vi "Get Errors.vi"(8 "error in (no error)":errorcluster, 10 "Parse All":bool, 11 "Plugin Manager in":refnum<class "CIFPluginManager.lvclass">) -> (0 "error out":errorcluster, 2 "Errors":T1[](array[typedef]), 3 "Plugin Manager out":refnum<class "CIFPluginManager.lvclass">)   [LabVIEW 2021, in "CIFPluginManager.lvclass"]
uses:
  CIFPluginManager.lvclass
  <vilib>/CIF Foundation/CIF Core/CIFUtilities/CIFLogs/Typedef/Error Message.ctl
  CIFPluginManager.lvclass/CIFPluginManager.ctl
  <vilib>/CIF Foundation/CIF Core/CIFUtilities/CIFLogs/CIFLogs.lvlib
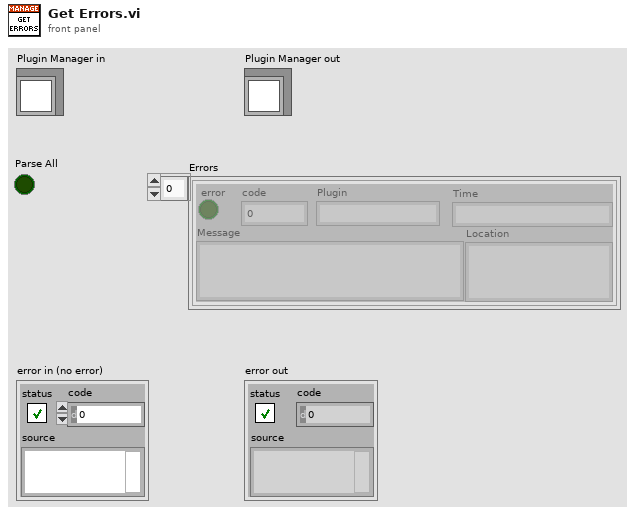
[diagram p1: front panel]
types:
  T1 = typedef "CIFLogs.lvlib/Error Message.ctl" = cluster{"error":bool, "code":i32, "Message":string, "Location":string, "Plugin":string, "Time":string}
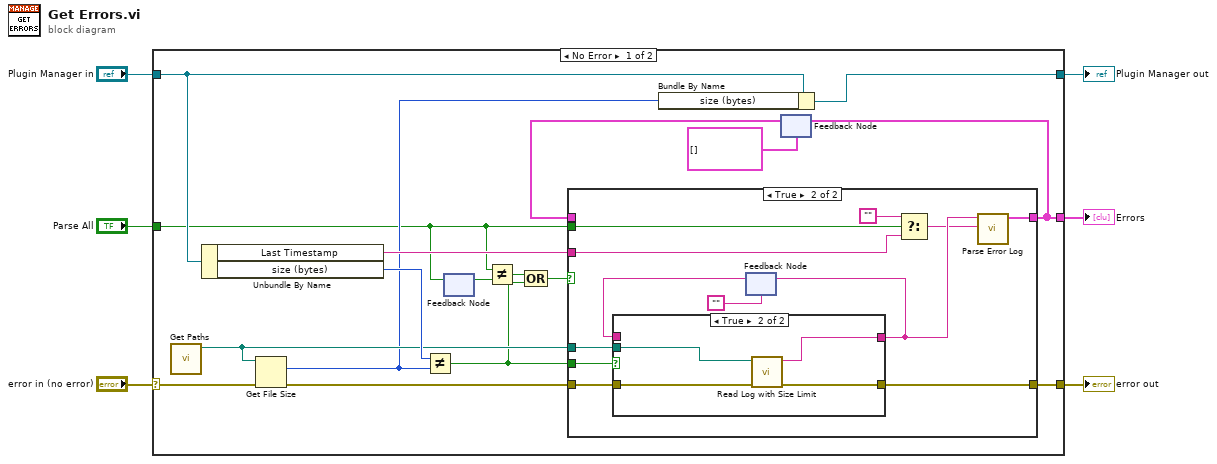
[diagram p0: block diagram]
diagram:
  n1 = case shown="No Error" "error in (no error)" {
    selector: "error in (no error)" -> [w18 w45]
    tunnel: [w23 w45] -> w1
    tunnel: [w19 w44] -> w3
    tunnel: "Plugin Manager in" -> [w20 w44]
    tunnel: [w9 _] -> w2
    tunnel: "Parse All" -> [w13 _]
    frame No Error {
      n2 = call <vilib>:"Get Paths.vi"() -> ("Error Log"=w17:path)  [unwired: 9 in, 2 out]
      n3 = Unbundle By Name(w20) -> ("Last Timestamp"=w21:string, "size (bytes)"=w22:i64)
      n4 = Get File Size(file=w17, error in=w18) -> (size (in bytes)=w15:i64, 0:w16:errorcluster)  [unwired: 1 out]
      n5 = Not Equal?(x=w22, y=w15) -> (x != y?=w11:bool)
      n6 = feedback-in #1(w13) -> ()
      n7 = feedback #1() -> (w14:bool)  [unwired: 1 in]
      n8 = Not Equal?(x=w13, y=w14) -> (x != y?=w12:bool)
      n9 = Compound Arithmetic op=OR(w12, w11) -> (w10:bool)
      n10 = Bundle By Name(cluster=w20, "size (bytes)"=w15) -> (w19:refnum<class "CIFPluginManager.lvclass">)
      n11 = feedback #2(T1[] [] ("Errors")) -> (w8:T1[])
      n12 = case shown="True" w10 {
        tunnel: [w24 w37] -> w23
        tunnel: [w25 w31] -> w9
        tunnel: w21 -> [_ w30]
        tunnel: w17 -> [_ w29]
        tunnel: w16 -> [w24 w28]
        tunnel: w13 -> [_ w27]
        tunnel: w11 -> [_ w26]
        tunnel: w8 -> [w25 _]
        frame False {
        }
        frame True {
          n13 = feedback #3("") -> (w34:string)
          n14 = case shown="True" w26 {
            tunnel: [w38 w40] -> w37
            tunnel: w29 -> [_ w42]
            tunnel: w28 -> [w38 w43]
            tunnel: [w39 w41] -> w33
            tunnel: w34 -> [w39 _]
            frame False {
            }
            frame True {
              n15 = call "Read Log with Size Limit.vi"("error in (no error)"=w43, "Info Log"=w42) -> ("error out"=w40:errorcluster, "Log"=w41:string)  [unwired: 8 in]
            }
          }
          n16 = feedback-in #3(w33) -> ()
          n17 = Select(t="", s=w27, f=w30) -> (s? t:f=w32:string)
          n18 = call <vilib>:"Parse Error Log.vi"("Index Timestamp"=w32, "Error Log"=w33) -> ("Errors"=w31:T1[])  [unwired: 9 in]
        }
      }
      n19 = feedback-in #2(w9) -> ()
    }
    frame Error {
    }
  }
  "error out" <- w1
  "Plugin Manager out" <- w3
  "Errors" <- w2
